vi "8X.vi"(0 "xml path":path=path "D:/wmgxml.xml", 1 "type":T4(ring)=enum."QSFP28", 5 "txtPath":path, 7 "singleItemInfo":T3[](array[typedef]), 9 "xml_detail":T1, 11 "TDD":T2, 12 "StatusRef":refnum<vi>) -> ()   [LabVIEW 2011]
uses:
  dataType/sSpec.ctl
  dataType/TDD.ctl
  dataType/xml_detail.ctl
panel:
  out "2nd":string
  out "cycle item names":string[](array[string])
  out "midVar_time":string[](array[string])
  out "cycle items":string[](array[string])
  out "Terminat Points":dbl[](array[numeric])
  out "TDD spec cable":string
  out "TDD spec terminal":string
  out "Cable Points":dbl[](array[numeric])
  out "TestResult":string
  out "input_array_time":string[](array[string])
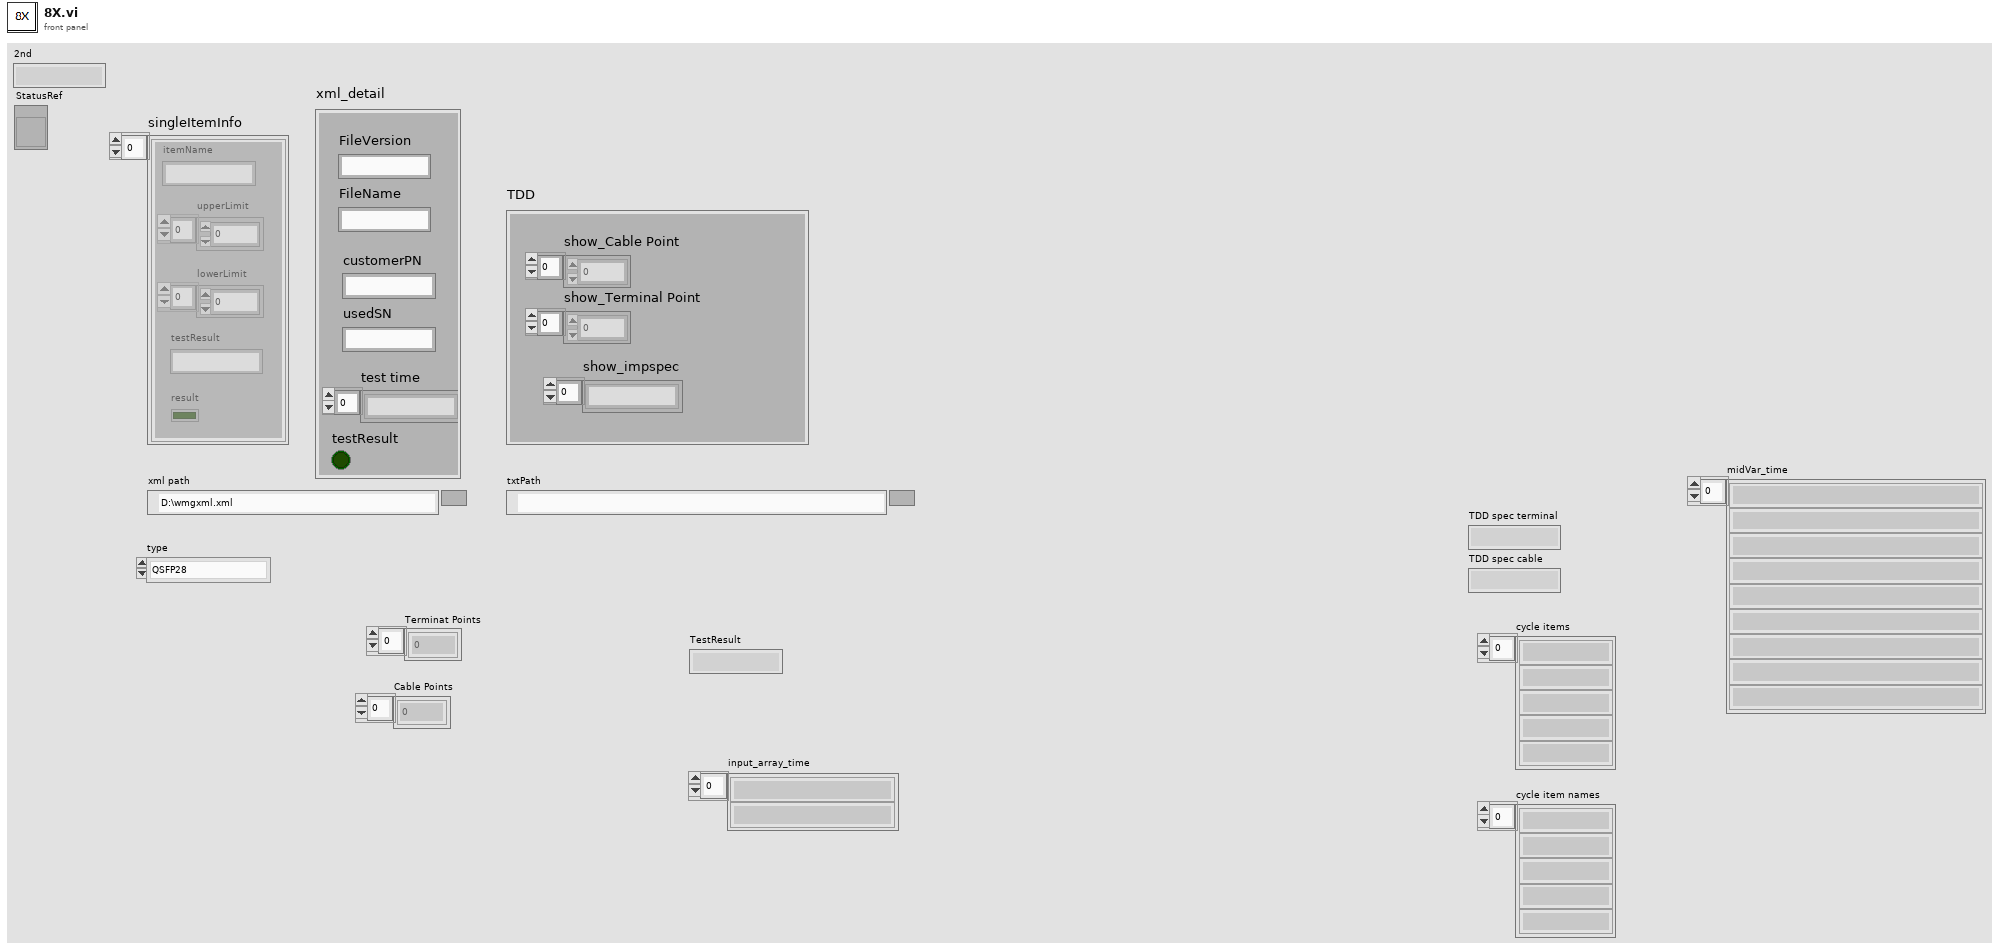
[diagram p1: front panel]
types:
  T1 = typedef "xml_detail.ctl" = cluster{"FileVersion":string, "FileName":string, "customerPN":string, "usedSN":string, "test time":string[], "testResult":bool}
  T2 = typedef "TDD.ctl" = cluster{"show_Cable Point":dbl[], "show_Terminal Point":dbl[], "show_impspec":string[]}
  T3 = typedef "sSpec.ctl" = cluster{"itemName":string, "upperLimit":dbl[], "lowerLimit":dbl[], "testResult":string, "result":bool}
  T4 = enum16{"MINI SAS HD 4X", "MINI SAS 4X", "SFP28", "QSFP28", "SFP+", "SLIM"}
  T5 = enum16{"open", "replace", "create", "open or create", "replace or create", "replace or create with confirmation"}
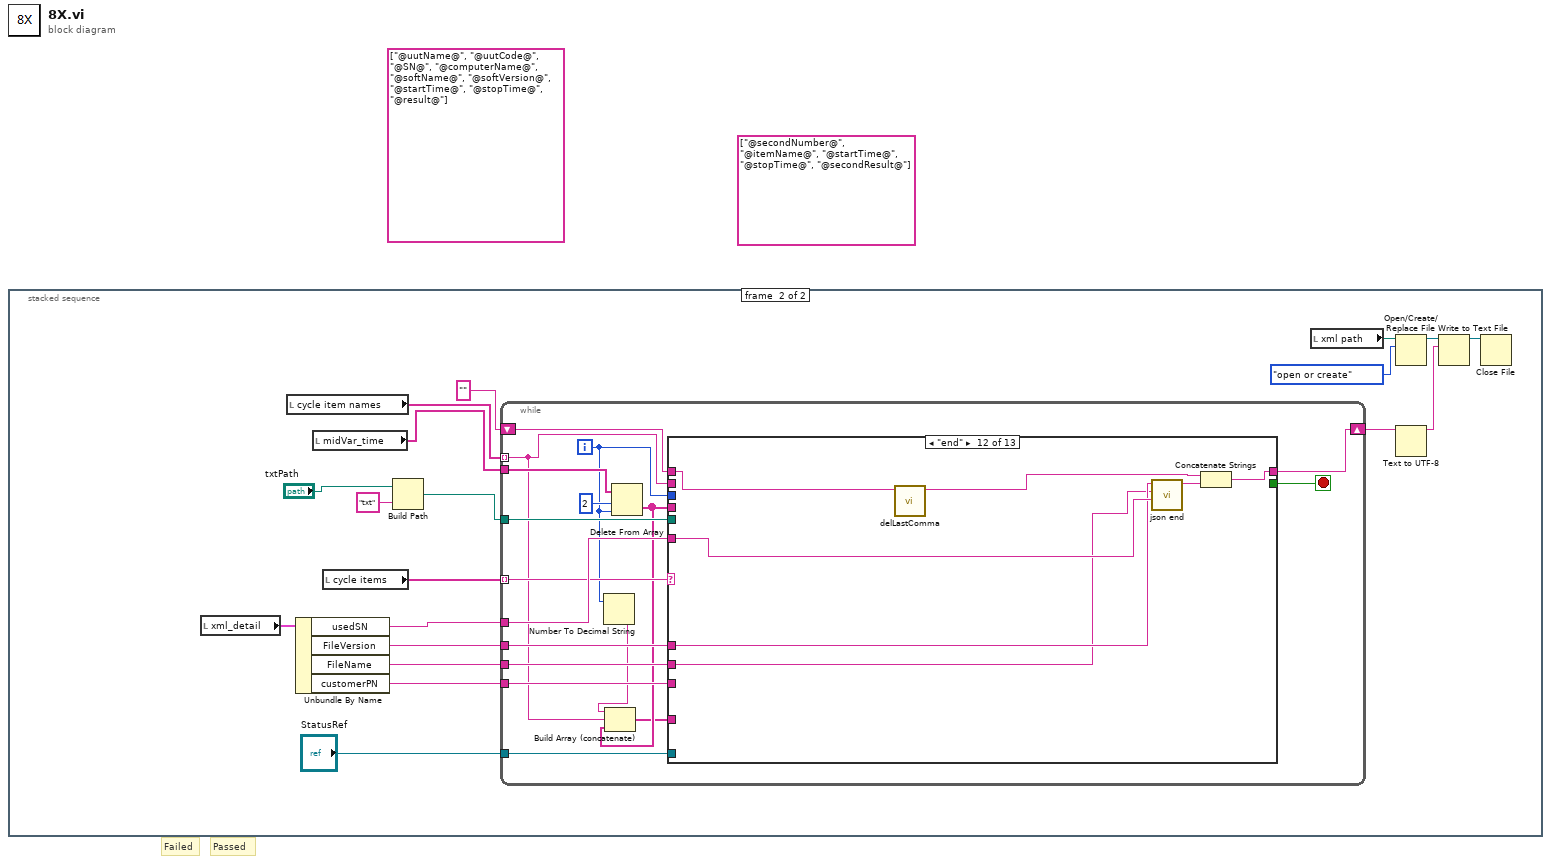
[diagram p0: block diagram]
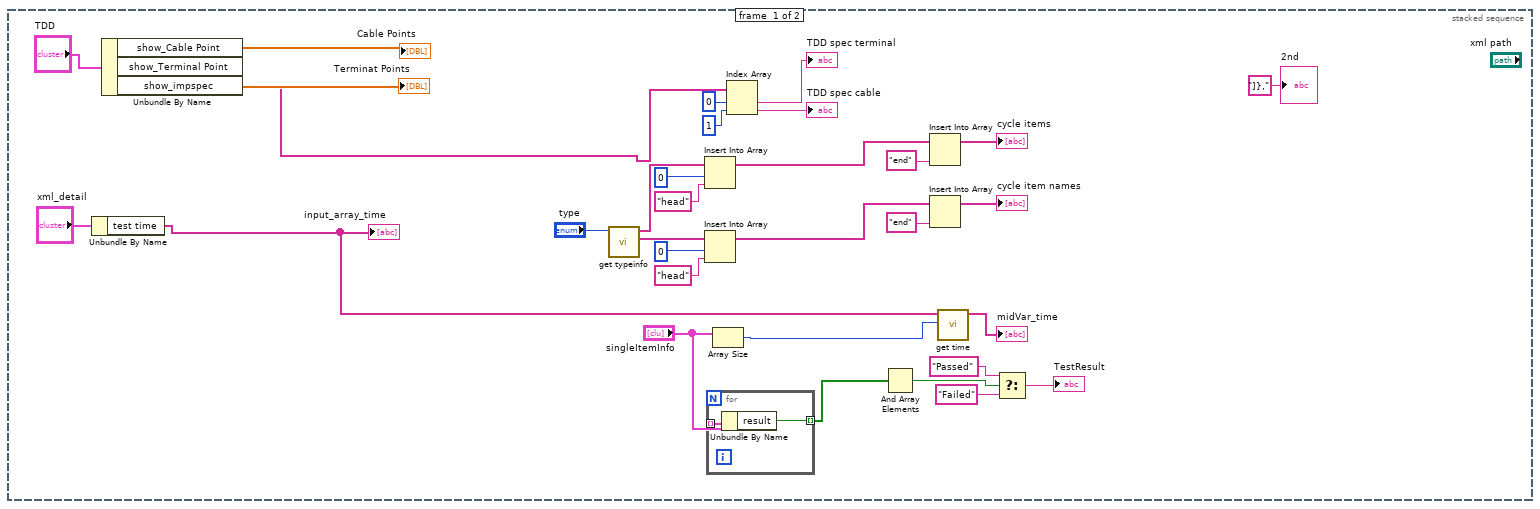
[diagram p2: hidden frame]
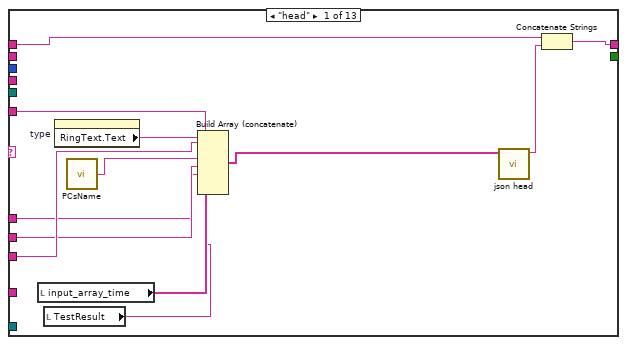
[diagram p3: hidden frame]
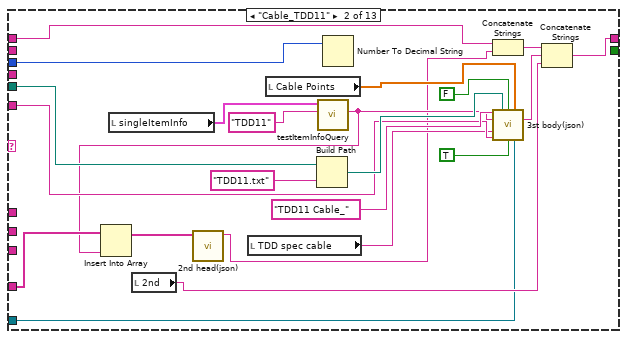
[diagram p4: hidden frame]
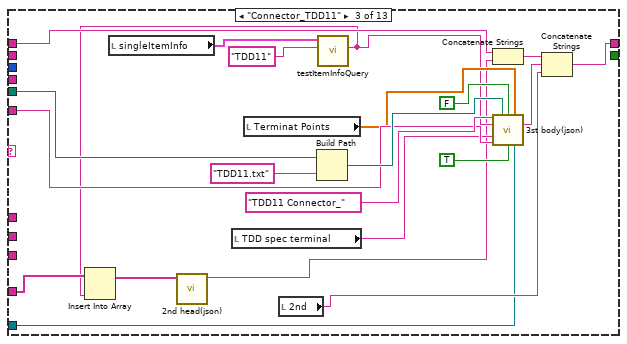
[diagram p5: hidden frame]
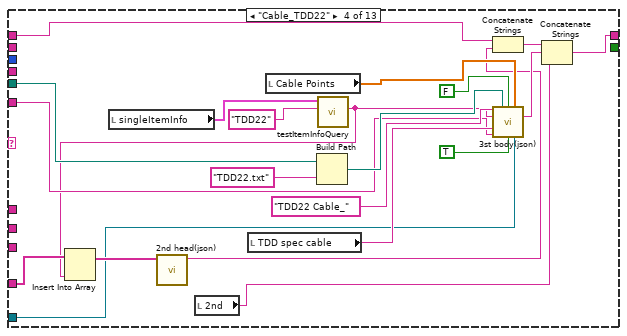
[diagram p6: hidden frame]
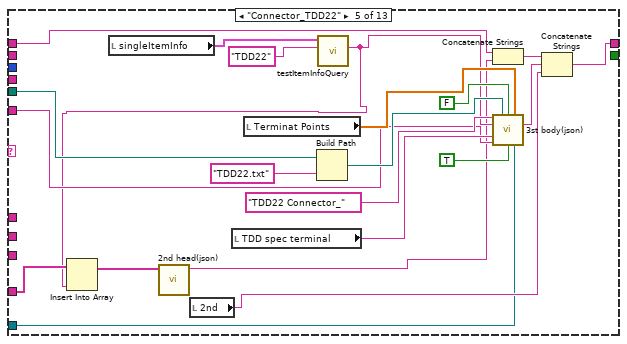
[diagram p7: hidden frame]
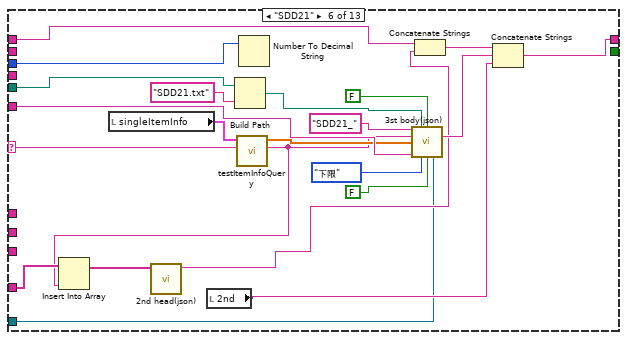
[diagram p8: hidden frame]
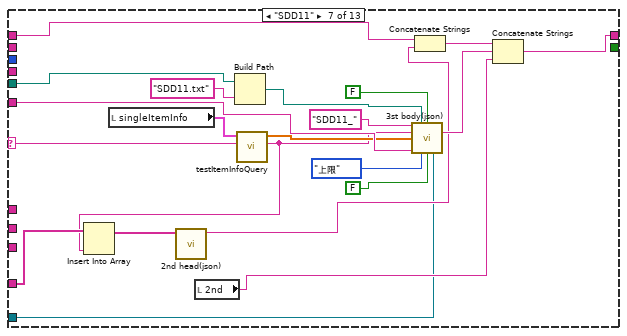
[diagram p9: hidden frame]
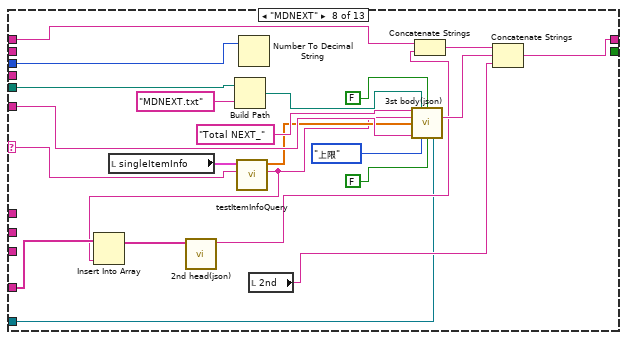
[diagram p10: hidden frame]
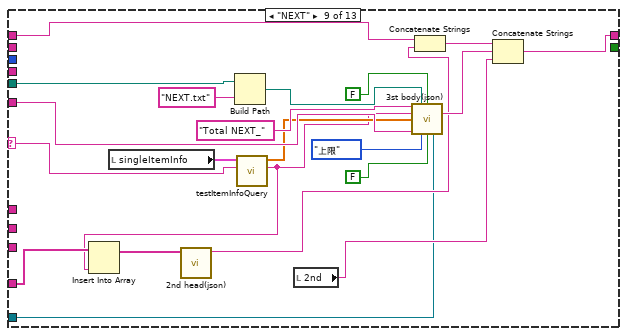
[diagram p11: hidden frame]
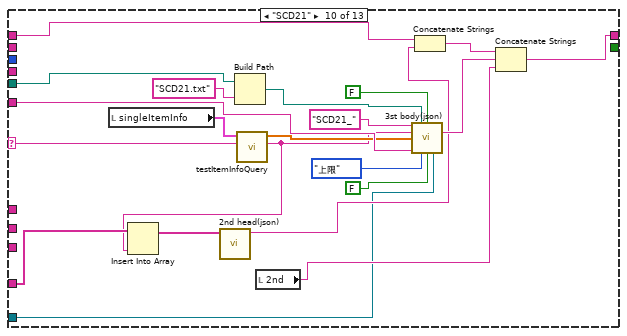
[diagram p12: hidden frame]
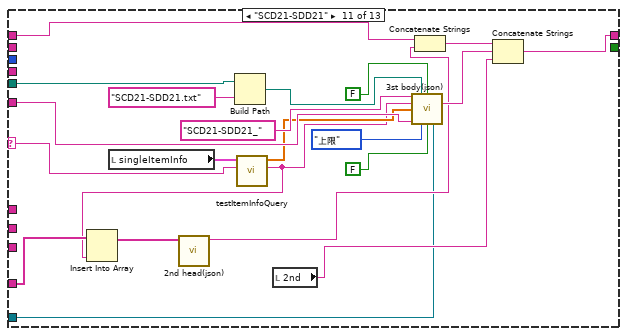
[diagram p13: hidden frame]
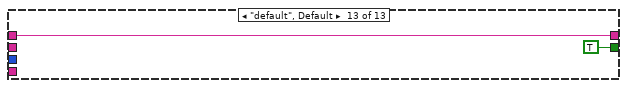
[diagram p14: hidden frame]
diagram:
  (unwired) string[] ["@uutName@", "@uutCode@", "@SN@", "@computerName@", "@softName@", "@softVersion@", "@startTime@", "@stopTime@", "@result@"]
  (unwired) string[] ["@secondNumber@", "@itemName@", "@startTime@", "@stopTime@", "@secondResult@"]
  # "Failed"
  # "Passed"
  n1 = stacked-sequence {
    frame #0 {
      n2 = Unbundle By Name("xml_detail") -> ("test time"=w2:string[])
      "input_array_time" <- w2
      n3 = Unbundle By Name("TDD") -> ("show_Cable Point"=→"Cable Points":dbl[], "show_Terminal Point"=→"Terminat Points":dbl[], "show_impspec"=w4:string[])
      n4 = call "get typeinfo.vi"("type"="type") -> ("second item names"=w16:string[], "test items"=w17:string[])  [unwired: 9 in]
      n5 = Insert Into Array(array=w17, index=0 ("索引"), new element="head" ("新元素/子数组")) -> (w26:string[])
      n6 = Insert Into Array(array=w16, index=0 ("索引"), new element="head" ("新元素/子数组")) -> (w20:string[])
      n7 = for {
        tunnel: "singleItemInfo" -> [w34] mode=indexing
        tunnel: [w33] -> w8 mode=indexing
        n8 = Unbundle By Name(w34) -> ("result"=w33:bool)
      }
      n9 = Array Size(array="singleItemInfo") -> (size(s)=w10:i32)
      n10 = Index Array(array=w4, index #1=0 ("索引"), index #2=1 ("索引")) -> (element #1=→"TDD spec terminal":string, element #2=→"TDD spec cable":string)
      n11 = And Array Elements(Boolean array=w8) -> (logical AND=w12:bool)
      n12 = Insert Into Array(array=w26, new element="end" ("新元素/子数组")) -> (→"cycle items":string[])  [unwired: 1 in]
      n13 = Insert Into Array(array=w20, new element="end" ("新元素/子数组")) -> (→"cycle item names":string[])  [unwired: 1 in]
      n14 = call "get time.vi"("item count"=w10, "input_array_time"=w2) -> ("midVar_time"=→"midVar_time":string[])  [unwired: 9 in]
      n15 = Select(t="Passed", s=w12, f="Failed") -> (s? t:f=→"TestResult":string)
      "2nd" <- "]}," ("字符串")
    }
    frame #1 {
      n16 = local read "xml_detail"() -> (w40:T1)
      n17 = local read "cycle item names"() -> (w44:string[])
      n18 = Unbundle By Name(w40) -> ("usedSN"=w39:string, "FileVersion"=w38:string, "FileName"=w37:string, "customerPN"=w36:string)
      n19 = local read "midVar_time"() -> (w45:string[])
      n20 = local read "cycle items"() -> (w52:string[])
      n21 = Build Path(base path="txtPath", name or relative path="txt" ("名称或相对路径")) -> (appended path=w41:path)
      n22 = while {
        tunnel: w52 -> [w65] mode=indexing
        shift-right: [w69] -> w47
        shift-left: "" -> [w70]
        tunnel: w41 -> [w68]
        tunnel: w39 -> [w67]
        tunnel: w45 -> [w64]
        tunnel: w44 -> [w57] mode=indexing
        tunnel: w38 -> [w62]
        tunnel: w37 -> [w61]
        tunnel: w36 -> [w60]
        tunnel: "StatusRef" -> [w54]
        i -> [w59]
        stop <- w66 stop-if-true
        n23 = Number To Decimal String(number=w59) -> (decimal integer string=w58:string)  [unwired: 1 in]
        n24 = Delete From Array(array=w64, length=2 ("长度"), index=w59) -> (deleted portion=w56:string[])  [unwired: 1 out]
        n25 = Build Array (concatenate)(w58, w57, w56) -> (w55:string[])
        n26 = case shown="\"end\"" w65 {
          selector: w65 -> [_ _ _ _ _ w174 w196 w217 w239 w260 w281 _ _]
          tunnel: w70 -> [w82 w103 w125 w146 w167 w188 w210 w231 w253 w274 w295 w297 w304]
          tunnel: [w81 w101 w123 w144 w165 w186 w208 w229 w251 w272 w293 w301 w304] -> w69
          tunnel: w59 -> [_ w104 _ _ _ w189 _ w232 _ _ _ _ _]
          tunnel: w68 -> [_ w98 w120 w141 w162 w183 w205 w226 w248 w269 w290 _ _]
          tunnel: w67 -> [w77 w93 w115 w134 w155 w178 w200 w221 w243 w264 w285 w300 _]
          tunnel: [_ _ _ _ _ _ _ _ _ _ _ _ TRUE] -> w66
          tunnel: w56 -> [_ _ _ _ _ _ _ _ _ _ _ _ _]
          tunnel: w57 -> [_ _ _ _ _ _ _ _ _ _ _ _ _]
          tunnel: w62 -> [w74 _ _ _ _ _ _ _ _ _ _ w299 _]
          tunnel: w61 -> [w75 _ _ _ _ _ _ _ _ _ _ w298 _]
          tunnel: w60 -> [w78 _ _ _ _ _ _ _ _ _ _ _ _]
          tunnel: w55 -> [_ w88 w109 w130 w151 w172 w194 w215 w237 w258 w279 _ _]
          tunnel: w54 -> [_ w83 w105 w126 w147 w168 w190 w211 w233 w254 w275 _ _]
          frame "head" {
            n27 = local read "input_array_time"() -> (w73:string[])
            n28 = local read "TestResult"() -> (w72:string)
            n29 = property on="type" class="Enum (严格)"() -> ("RingText.Text"=w79:string)  [unwired: 2 in, 2 out]
            n30 = call "PCsName.vi"() -> ("Computer Name"=w76:string)
            n31 = Build Array (concatenate)(w79, w78, w77, w76, w75, w74, w73, w72) -> (w71:string[])
            n32 = call "json head.vi"("information"=w71) -> ("midVar_Content"=w80:string)  [unwired: 10 in]
            n33 = Concatenate Strings(w82, w80) -> (w81:string)
          }
          frame "Cable_TDD11" {
            n34 = local read "singleItemInfo"() -> (w90:T3[])
            n35 = local read "2nd"() -> (w84:string)
            n36 = local read "TDD spec cable"() -> (w92:string)
            n37 = local read "Cable Points"() -> (w91:dbl[])
            n38 = Build Path(base path=w98, name or relative path="TDD11.txt" ("名称或相对路径")) -> (appended path=w96:path)
            n39 = call "testItemInfoQuery.vi"("testItem"="TDD11" ("test item"), "singleItemInfo"=w90) -> ("testResult"=w86:string)  [unwired: 8 in, 1 out]
            n40 = Insert Into Array(array=w88, new element=w86) -> (w87:string[])  [unwired: 1 in]
            n41 = call "2nd head(json).vi"("value"=w87) -> ("midVar_Content"=w85:string)  [unwired: 10 in]
            n42 = Number To Decimal String(number=w104) -> ()  [unwired: 1 in, 1 out]
            n43 = Concatenate Strings(w103, w85) -> (w102:string)
            n44 = call "3st body(json).vi"("third test item name"="TDD11 Cable_", "file path (dialog if empty)"=w96, "ABS?"=FALSE, "Points"=w91, "second result"=w86, "TDD spec"=w92, "SN"=w93, "TDD?"=TRUE, "StatusRef"=w83) -> ("OutPutXml"=w100:string)  [unwired: 6 in]
            n45 = Concatenate Strings(w102, w100, w84) -> (w101:string)
          }
          frame "Connector_TDD11" {
            n46 = local read "singleItemInfo"() -> (w112:T3[])
            n47 = local read "TDD spec terminal"() -> (w113:string)
            n48 = local read "Terminat Points"() -> (w114:dbl[])
            n49 = local read "2nd"() -> (w106:string)
            n50 = Build Path(base path=w120, name or relative path="TDD11.txt" ("名称或相对路径")) -> (appended path=w118:path)
            n51 = call "testItemInfoQuery.vi"("testItem"="TDD11" ("test item"), "singleItemInfo"=w112) -> ("testResult"=w108:string)  [unwired: 8 in, 1 out]
            n52 = Insert Into Array(array=w109, new element=w108) -> (w110:string[])  [unwired: 1 in]
            n53 = call "2nd head(json).vi"("value"=w110) -> ("midVar_Content"=w107:string)  [unwired: 10 in]
            n54 = Concatenate Strings(w125, w107) -> (w124:string)
            n55 = call "3st body(json).vi"("third test item name"="TDD11 Connector_", "file path (dialog if empty)"=w118, "ABS?"=FALSE, "Points"=w114, "second result"=w108, "TDD spec"=w113, "SN"=w115, "TDD?"=TRUE, "StatusRef"=w105) -> ("OutPutXml"=w122:string)  [unwired: 6 in]
            n56 = Concatenate Strings(w124, w122, w106) -> (w123:string)
          }
          frame "Cable_TDD22" {
            n57 = local read "singleItemInfo"() -> (w133:T3[])
            n58 = local read "2nd"() -> (w127:string)
            n59 = local read "TDD spec cable"() -> (w135:string)
            n60 = local read "Cable Points"() -> (w136:dbl[])
            n61 = Build Path(base path=w141, name or relative path="TDD22.txt" ("名称或相对路径")) -> (appended path=w139:path)
            n62 = call "testItemInfoQuery.vi"("testItem"="TDD22" ("test item"), "singleItemInfo"=w133) -> ("testResult"=w129:string)  [unwired: 8 in, 1 out]
            n63 = Insert Into Array(array=w130, new element=w129) -> (w131:string[])  [unwired: 1 in]
            n64 = call "2nd head(json).vi"("value"=w131) -> ("midVar_Content"=w128:string)  [unwired: 10 in]
            n65 = Concatenate Strings(w146, w128) -> (w145:string)
            n66 = call "3st body(json).vi"("third test item name"="TDD22 Cable_", "file path (dialog if empty)"=w139, "ABS?"=FALSE, "Points"=w136, "second result"=w129, "TDD spec"=w135, "SN"=w134, "TDD?"=TRUE, "StatusRef"=w126) -> ("OutPutXml"=w143:string)  [unwired: 6 in]
            n67 = Concatenate Strings(w145, w143, w127) -> (w144:string)
          }
          frame "Connector_TDD22" {
            n68 = local read "singleItemInfo"() -> (w154:T3[])
            n69 = local read "2nd"() -> (w148:string)
            n70 = local read "TDD spec terminal"() -> (w156:string)
            n71 = local read "Terminat Points"() -> (w157:dbl[])
            n72 = Build Path(base path=w162, name or relative path="TDD22.txt" ("名称或相对路径")) -> (appended path=w160:path)
            n73 = call "testItemInfoQuery.vi"("testItem"="TDD22" ("test item"), "singleItemInfo"=w154) -> ("testResult"=w150:string)  [unwired: 8 in, 1 out]
            n74 = Insert Into Array(array=w151, new element=w150) -> (w152:string[])  [unwired: 1 in]
            n75 = call "2nd head(json).vi"("value"=w152) -> ("midVar_Content"=w149:string)  [unwired: 10 in]
            n76 = Concatenate Strings(w167, w149) -> (w166:string)
            n77 = call "3st body(json).vi"("third test item name"="TDD22 Connector_", "file path (dialog if empty)"=w160, "ABS?"=FALSE, "Points"=w157, "second result"=w150, "TDD spec"=w156, "SN"=w155, "TDD?"=TRUE, "StatusRef"=w147) -> ("OutPutXml"=w164:string)  [unwired: 6 in]
            n78 = Concatenate Strings(w166, w164, w148) -> (w165:string)
          }
          frame "SDD21" {
            n79 = local read "singleItemInfo"() -> (w176:T3[])
            n80 = local read "2nd"() -> (w169:string)
            n81 = Build Path(base path=w183, name or relative path="SDD21.txt" ("名称或相对路径")) -> (appended path=w181:path)
            n82 = call "testItemInfoQuery.vi"("testItem"=w174, "singleItemInfo"=w176) -> ("testResult"=w171:string, "Limit"=w175:dbl[])  [unwired: 8 in]
            n83 = Insert Into Array(array=w172, new element=w171) -> (w173:string[])  [unwired: 1 in]
            n84 = call "2nd head(json).vi"("value"=w173) -> ("midVar_Content"=w170:string)  [unwired: 10 in]
            n85 = Number To Decimal String(number=w189) -> ()  [unwired: 1 in, 1 out]
            n86 = call "3st body(json).vi"("third test item name"="SDD21_", "file path (dialog if empty)"=w181, "ABS?"=FALSE, "second result"=w171, "single spec"=w175, "SN"=w178, "limit type"=enum16{"上限", "下限"}."下限", "TDD?"=FALSE, "StatusRef"=w168) -> ("OutPutXml"=w185:string)  [unwired: 6 in]
            n87 = Concatenate Strings(w188, w170) -> (w187:string)
            n88 = Concatenate Strings(w187, w185, w169) -> (w186:string)
          }
          frame "SDD11" {
            n89 = local read "singleItemInfo"() -> (w198:T3[])
            n90 = local read "2nd"() -> (w191:string)
            n91 = Build Path(base path=w205, name or relative path="SDD11.txt" ("名称或相对路径")) -> (appended path=w203:path)
            n92 = call "testItemInfoQuery.vi"("testItem"=w196, "singleItemInfo"=w198) -> ("testResult"=w193:string, "Limit"=w197:dbl[])  [unwired: 8 in]
            n93 = Insert Into Array(array=w194, new element=w193) -> (w195:string[])  [unwired: 1 in]
            n94 = call "2nd head(json).vi"("value"=w195) -> ("midVar_Content"=w192:string)  [unwired: 10 in]
            n95 = call "3st body(json).vi"("third test item name"="SDD11_", "file path (dialog if empty)"=w203, "ABS?"=FALSE, "second result"=w193, "single spec"=w197, "SN"=w200, "limit type"=enum16{"上限", "下限"}."上限", "TDD?"=FALSE, "StatusRef"=w190) -> ("OutPutXml"=w207:string)  [unwired: 6 in]
            n96 = Concatenate Strings(w210, w192) -> (w209:string)
            n97 = Concatenate Strings(w209, w207, w191) -> (w208:string)
          }
          frame "MDNEXT" {
            n98 = local read "singleItemInfo"() -> (w219:T3[])
            n99 = Build Path(base path=w226, name or relative path="MDNEXT.txt" ("名称或相对路径")) -> (appended path=w224:path)
            n100 = call "testItemInfoQuery.vi"("testItem"=w217, "singleItemInfo"=w219) -> ("testResult"=w214:string, "Limit"=w218:dbl[])  [unwired: 8 in]
            n101 = Insert Into Array(array=w215, new element=w214) -> (w216:string[])  [unwired: 1 in]
            n102 = call "2nd head(json).vi"("value"=w216) -> ("midVar_Content"=w213:string)  [unwired: 10 in]
            n103 = Number To Decimal String(number=w232) -> ()  [unwired: 1 in, 1 out]
            n104 = local read "2nd"() -> (w212:string)
            n105 = call "3st body(json).vi"("third test item name"="Total NEXT_", "file path (dialog if empty)"=w224, "ABS?"=FALSE, "second result"=w214, "single spec"=w218, "SN"=w221, "limit type"=enum16{"上限", "下限"}."上限", "TDD?"=FALSE, "StatusRef"=w211) -> ("OutPutXml"=w228:string)  [unwired: 6 in]
            n106 = Concatenate Strings(w231, w213) -> (w230:string)
            n107 = Concatenate Strings(w230, w228, w212) -> (w229:string)
          }
          frame "NEXT" {
            n108 = local read "singleItemInfo"() -> (w241:T3[])
            n109 = Build Path(base path=w248, name or relative path="NEXT.txt" ("名称或相对路径")) -> (appended path=w246:path)
            n110 = call "testItemInfoQuery.vi"("testItem"=w239, "singleItemInfo"=w241) -> ("testResult"=w236:string, "Limit"=w240:dbl[])  [unwired: 8 in]
            n111 = Insert Into Array(array=w237, new element=w236) -> (w238:string[])  [unwired: 1 in]
            n112 = call "2nd head(json).vi"("value"=w238) -> ("midVar_Content"=w235:string)  [unwired: 10 in]
            n113 = local read "2nd"() -> (w234:string)
            n114 = call "3st body(json).vi"("third test item name"="Total NEXT_", "file path (dialog if empty)"=w246, "ABS?"=FALSE, "second result"=w236, "single spec"=w240, "SN"=w243, "limit type"=enum16{"上限", "下限"}."上限", "TDD?"=FALSE, "StatusRef"=w233) -> ("OutPutXml"=w250:string)  [unwired: 6 in]
            n115 = Concatenate Strings(w253, w235) -> (w252:string)
            n116 = Concatenate Strings(w252, w250, w234) -> (w251:string)
          }
          frame "SCD21" {
            n117 = local read "singleItemInfo"() -> (w262:T3[])
            n118 = Build Path(base path=w269, name or relative path="SCD21.txt" ("名称或相对路径")) -> (appended path=w267:path)
            n119 = call "testItemInfoQuery.vi"("testItem"=w260, "singleItemInfo"=w262) -> ("testResult"=w257:string, "Limit"=w261:dbl[])  [unwired: 8 in]
            n120 = Insert Into Array(array=w258, new element=w257) -> (w259:string[])  [unwired: 1 in]
            n121 = call "2nd head(json).vi"("value"=w259) -> ("midVar_Content"=w256:string)  [unwired: 10 in]
            n122 = local read "2nd"() -> (w255:string)
            n123 = call "3st body(json).vi"("third test item name"="SCD21_", "file path (dialog if empty)"=w267, "ABS?"=FALSE, "second result"=w257, "single spec"=w261, "SN"=w264, "limit type"=enum16{"上限", "下限"}."上限", "TDD?"=FALSE, "StatusRef"=w254) -> ("OutPutXml"=w271:string)  [unwired: 6 in]
            n124 = Concatenate Strings(w274, w256) -> (w273:string)
            n125 = Concatenate Strings(w273, w271, w255) -> (w272:string)
          }
          frame "SCD21-SDD21" {
            n126 = local read "singleItemInfo"() -> (w283:T3[])
            n127 = Build Path(base path=w290, name or relative path="SCD21-SDD21.txt" ("名称或相对路径")) -> (appended path=w288:path)
            n128 = call "testItemInfoQuery.vi"("testItem"=w281, "singleItemInfo"=w283) -> ("testResult"=w278:string, "Limit"=w282:dbl[])  [unwired: 8 in]
            n129 = Insert Into Array(array=w279, new element=w278) -> (w280:string[])  [unwired: 1 in]
            n130 = call "2nd head(json).vi"("value"=w280) -> ("midVar_Content"=w277:string)  [unwired: 10 in]
            n131 = local read "2nd"() -> (w276:string)
            n132 = call "3st body(json).vi"("third test item name"="SCD21-SDD21_", "file path (dialog if empty)"=w288, "ABS?"=FALSE, "second result"=w278, "single spec"=w282, "SN"=w285, "limit type"=enum16{"上限", "下限"}."上限", "TDD?"=FALSE, "StatusRef"=w275) -> ("OutPutXml"=w292:string)  [unwired: 6 in]
            n133 = Concatenate Strings(w295, w277) -> (w294:string)
            n134 = Concatenate Strings(w294, w292, w276) -> (w293:string)
          }
          frame "end" {
            n135 = call "delLastComma.vi"("字符串"=w297) -> ("result string"=w296:string)  [unwired: 10 in]
            n136 = call "json end.vi"("SN"=w300, "FilePath"=w298, "FileVer"=w299) -> ("midVar_Content"=w302:string)  [unwired: 8 in]
            n137 = Concatenate Strings(w296, w302) -> (w301:string)
          }
          frame "default", Default {
          }
        }
      }
      n138 = local read "xml path"() -> (w46:path)
      n139 = Open/Create/Replace File(file path (use dialog)=w46, operation (0:open)=T5."open or create" ("操作(0:open)")) -> (refnum out=w50:refnum<file>)  [unwired: 4 in, 2 out]
      n140 = Text to UTF-8(11:w47) -> (3:w48:string)  [unwired: 1 in, 1 out]
      n141 = Write to Text File(file (use dialog)=w50, text=w48) -> (refnum out=w49:refnum<file>)  [unwired: 2 in, 2 out]
      n142 = Close File(refnum=w49) -> ()  [unwired: 1 in, 2 out]
    }
  }
